vi "lab1_packet_formatter.vi"(8 "counter":i32, 9 "payload(bytes array)":u8[](array[numeric]), 11 "preamble(bytes array)":i16[](array[numeric])) -> (3 "bitstream":i16[](array[numeric]))   [LabVIEW 2014]
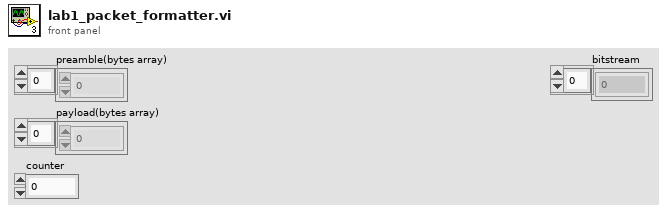
[diagram p1: front panel]
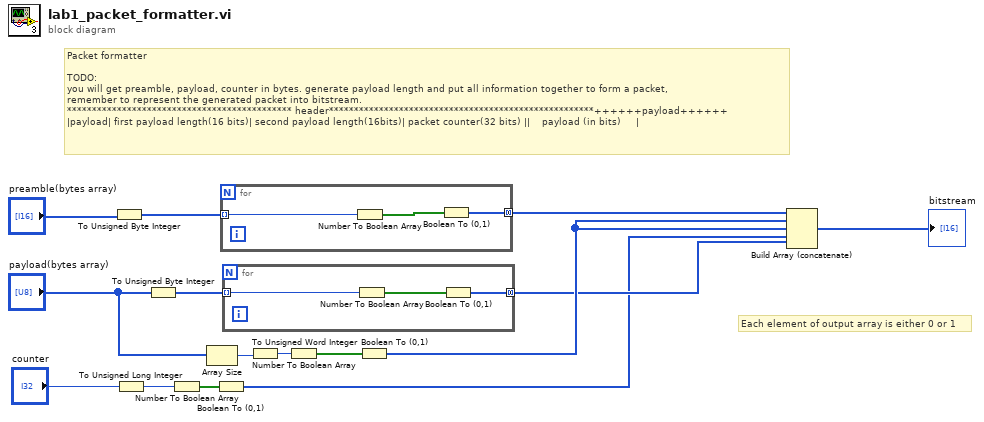
[diagram p0: block diagram]
diagram:
  # "Each element of output array is either 0 or 1"
  # "Packet formatter\n\nTODO: \nyou will get preamble, payload, counter in bytes. generate payload length and put all information together to form a packet, \nremember to represent the generated packet into bitstream. \n********************************************* header*****************************************************++++++payload++++++                  \n|payload| first payload length(16 bits)| second payload length(16bits)| packet counter(32 bits) ||    payload (in bits)     |"
  n1 = To Unsigned Byte Integer(number="preamble(bytes array)") -> (unsigned 8bit integer=w11:u8[])
  n2 = To Unsigned Long Integer(number="counter") -> (unsigned 32bit integer=w7:u32)
  n3 = To Unsigned Byte Integer(number="payload(bytes array)") -> (unsigned 8bit integer=w8:u8[])
  n4 = Number To Boolean Array(number=w7) -> (Boolean array=w6:bool[])
  n5 = Array Size(array="payload(bytes array)") -> (size(s)=w14:i32)
  n6 = Boolean To (0,1)(Boolean=w6) -> (0, 1=w1:i16[])
  n7 = for {
    tunnel: w11 -> [w16] mode=indexing
    tunnel: [w18] -> w5 mode=concatenating
    n8 = Number To Boolean Array(number=w16) -> (Boolean array=w17:bool[])
    n9 = Boolean To (0,1)(Boolean=w17) -> (0, 1=w18:i16[])
  }
  n10 = for {
    tunnel: [w21] -> w2 mode=concatenating
    tunnel: w8 -> [w19] mode=indexing
    n11 = Number To Boolean Array(number=w19) -> (Boolean array=w20:bool[])
    n12 = Boolean To (0,1)(Boolean=w20) -> (0, 1=w21:i16[])
  }
  n13 = To Unsigned Word Integer(number=w14) -> (unsigned 16bit integer=w13:u16)
  n14 = Number To Boolean Array(number=w13) -> (Boolean array=w15:bool[])
  n15 = Boolean To (0,1)(Boolean=w15) -> (0, 1=w3:i16[])
  n16 = Build Array (concatenate)(w5, w3, w3, w1, w2) -> (→"bitstream":i16[])
